vi "Get Perimeter Nodes.vi"(11 "Point":T1) -> (3 "Array":T1[](array[typedef]))   [LabVIEW 2023]
uses:
  Cluster_Point.ctl
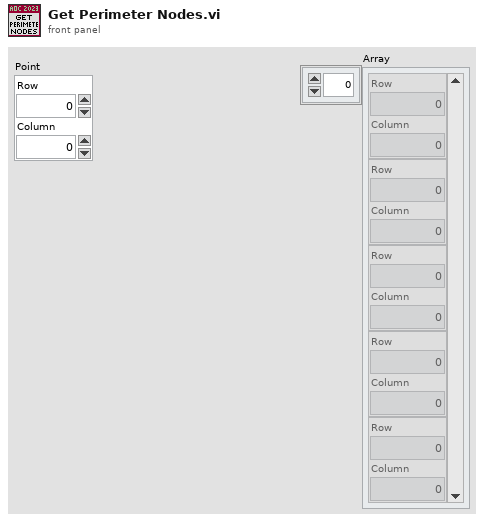
[diagram p1: front panel]
types:
  T1 = typedef "Cluster_Point.ctl" = cluster{"Row":i32, "Column":i32}
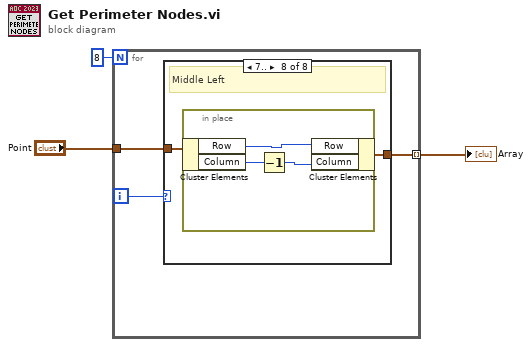
[diagram p0: block diagram]
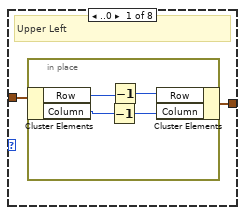
[diagram p2: hidden frame]
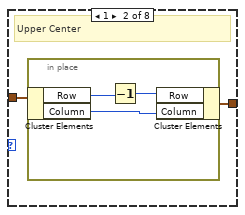
[diagram p3: hidden frame]
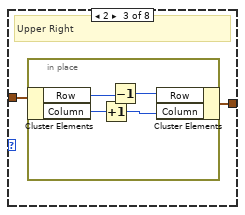
[diagram p4: hidden frame]
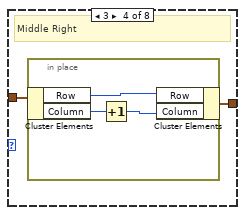
[diagram p5: hidden frame]
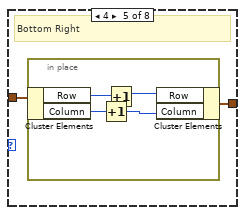
[diagram p6: hidden frame]
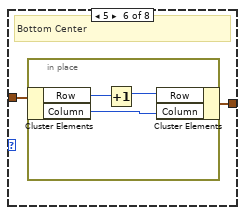
[diagram p7: hidden frame]
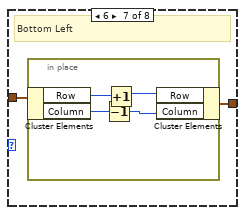
[diagram p8: hidden frame]
diagram:
  n1 = for {
    N: 8 -> [_]
    tunnel: "Point" -> [w5]
    tunnel: [w4] -> w1 mode=indexing
    i -> [w6]
    n2 = case shown="7.." w6 {
      tunnel: w5 -> [w8 w14 w19 w25 w30 w36 w41 w47]
      tunnel: [w7 w13 w18 w24 w29 w35 w40 w46] -> w4
      frame ..0 {
        # "Upper Left"
        n3 = in-place {
          n4 = in-place-cluster #1(w8) -> ("Row"=w12:i32, "Column"=w10:i32)
          n5 = Decrement(x=w10) -> (x-1=w9:i32)
          n6 = Decrement(x=w12) -> (x-1=w11:i32)
          n7 = in-place-cluster #1("Row"=w11, "Column"=w9) -> (w7:T1)
        }
      }
      frame 1 {
        # "Upper Center"
        n8 = in-place {
          n9 = in-place-cluster #2(w14) -> ("Row"=w17:i32, "Column"=w15:i32)
          n10 = Decrement(x=w17) -> (x-1=w16:i32)
          n11 = in-place-cluster #2("Row"=w16, "Column"=w15) -> (w13:T1)
        }
      }
      frame 2 {
        # "Upper Right"
        n12 = in-place {
          n13 = in-place-cluster #3(w19) -> ("Row"=w23:i32, "Column"=w21:i32)
          n14 = Increment(x=w21) -> (x+1=w20:i32)
          n15 = Decrement(x=w23) -> (x-1=w22:i32)
          n16 = in-place-cluster #3("Row"=w22, "Column"=w20) -> (w18:T1)
        }
      }
      frame 3 {
        # "Middle Right"
        n17 = in-place {
          n18 = in-place-cluster #4(w25) -> ("Row"=w26:i32, "Column"=w28:i32)
          n19 = Increment(x=w28) -> (x+1=w27:i32)
          n20 = in-place-cluster #4("Row"=w26, "Column"=w27) -> (w24:T1)
        }
      }
      frame 4 {
        # "Bottom Right"
        n21 = in-place {
          n22 = in-place-cluster #5(w30) -> ("Row"=w32:i32, "Column"=w34:i32)
          n23 = Increment(x=w34) -> (x+1=w33:i32)
          n24 = Increment(x=w32) -> (x+1=w31:i32)
          n25 = in-place-cluster #5("Row"=w31, "Column"=w33) -> (w29:T1)
        }
      }
      frame 5 {
        # "Bottom Center"
        n26 = in-place {
          n27 = in-place-cluster #6(w36) -> ("Row"=w39:i32, "Column"=w37:i32)
          n28 = Increment(x=w39) -> (x+1=w38:i32)
          n29 = in-place-cluster #6("Row"=w38, "Column"=w37) -> (w35:T1)
        }
      }
      frame 6 {
        # "Bottom Left"
        n30 = in-place {
          n31 = in-place-cluster #7(w41) -> ("Row"=w45:i32, "Column"=w43:i32)
          n32 = Decrement(x=w43) -> (x-1=w42:i32)
          n33 = Increment(x=w45) -> (x+1=w44:i32)
          n34 = in-place-cluster #7("Row"=w44, "Column"=w42) -> (w40:T1)
        }
      }
      frame 7.. {
        # "Middle Left"
        n35 = in-place {
          n36 = in-place-cluster #8(w47) -> ("Row"=w48:i32, "Column"=w50:i32)
          n37 = Decrement(x=w50) -> (x-1=w49:i32)
          n38 = in-place-cluster #8("Row"=w48, "Column"=w49) -> (w46:T1)
        }
      }
    }
  }
  "Array" <- w1
